vi "Read logger name.vi"(11 "Logger in":refnum<class "Logger.lvclass">) -> (2 "logger name":string="main", 3 "Logger out":refnum<class "Logger.lvclass">)   [LabVIEW 2017, in "Logger.lvclass"]
uses:
  Logger.lvclass
  Logger.lvclass/Logger.ctl
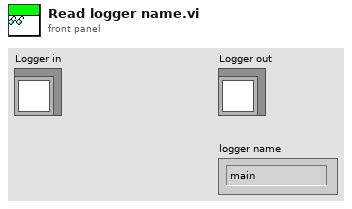
[diagram p1: front panel]
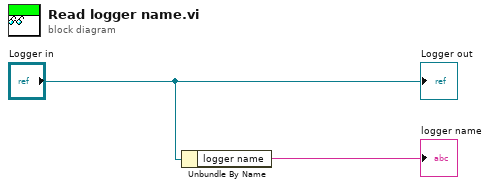
[diagram p0: block diagram]
diagram:
  n1 = Unbundle By Name("Logger in") -> ("logger name"=→"logger name":string)
  "Logger out" <- "Logger in"
